vi "Update-storage-file-prefix.vi"(8 "error in (no error)":errorcluster, 11 "Storage params. ref. in":refnum<data-value>) -> (0 "error out":errorcluster, 3 "Storage params. ref.":refnum<data-value>)   [LabVIEW 2013, in "CameraVision.lvlib" / "CV-Storage.lvclass"]
doc: "In case a separate file has to be saved for each acquisition iteration ('Storage mode' == \"1 file per layer\"), this VI adds a zero-padded iteration/layer number to the 'Base file name'.\n\nThe maximum supported layer number is 99 999 (= 100 000 layers).s"
uses:
  CV-Storage.lvclass
  CV-Storage.lvclass/CV-Storage.ctl
  Read Storage mode.vi
  Read Layer index.vi
  Read Base file name.vi
  Write Storage prefix.vi
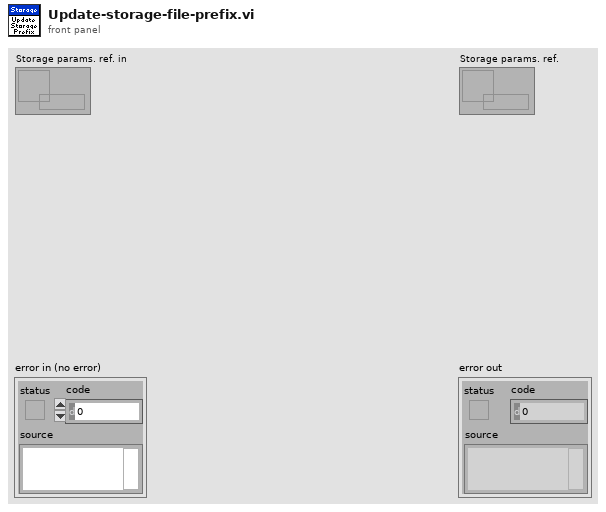
[diagram p1: front panel]
types:
  T1 = enum16{"1 file per layer", "1 file for all layers "}
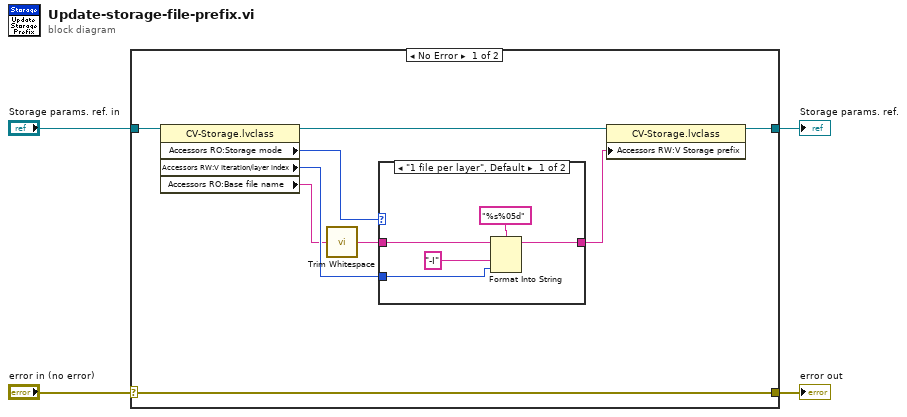
[diagram p0: block diagram]
diagram:
  n1 = case shown="No Error" "error in (no error)" {
    selector: "error in (no error)" -> [w13 w21]
    tunnel: [w13 w21] -> w3
    tunnel: [w10 w20] -> w1
    tunnel: "Storage params. ref. in" -> [w12 w20]
    frame No Error {
      n2 = property class="CV-Storage.lvclass"(reference=w12) -> (reference out=w9:refnum<data-value>, "Accessors RO:Storage mode"=w11:T1, "Accessors RW:V Iteration/layer index"=w8:u16, "Accessors RO:Base file name"=w7:string)  [unwired: 1 in, 1 out]
      n3 = call <vilib>:"Trim Whitespace.vi"("string"=w7) -> ("trimmed string"=w5:string)  [unwired: 1 in]
      n4 = case shown="\"1 file per layer\", Default" w11 {
        tunnel: w8 -> [w16 _]
        tunnel: [w15 w19] -> w6
        tunnel: w5 -> [w14 w19]
        frame "1 file per layer", Default {
          n5 = Format Into String(format string="%s%05d", initial string=w14, "-I", w16) -> (resulting string=w15:string)  [unwired: 1 in, 1 out]
        }
        frame "1 file for all layers " {
        }
      }
      n6 = property class="CV-Storage.lvclass"(reference=w9, "Accessors RW:V Storage prefix"=w6) -> (reference out=w10:refnum<data-value>)  [unwired: 1 in, 1 out]
    }
    frame Error {
    }
  }
  "error out" <- w3
  "Storage params. ref." <- w1
